vi "Data logger Default Paths.vi"(3 "Path Type":T1(ring)) -> (0 "Path":path)   [LabVIEW 2014]
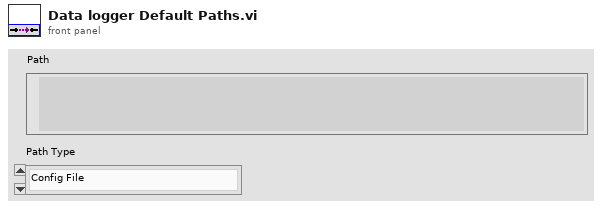
[diagram p1: front panel]
types:
  T1 = enum16{"Config File", "Image File", "Word Template", "Release Note", "Help HTML", "Help Word", "Error List", "Excel Template", "CSV Template", "Tray Icon"}
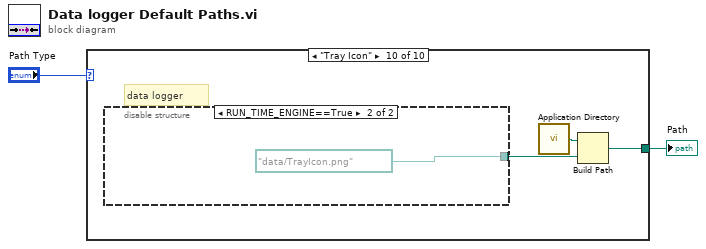
[diagram p0: block diagram]
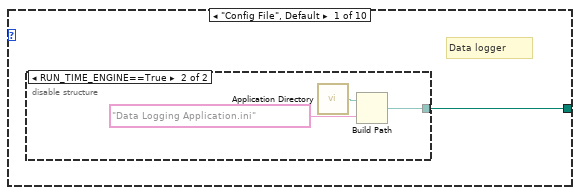
[diagram p2: hidden frame]
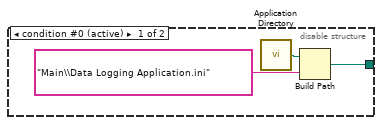
[diagram p3: hidden frame]
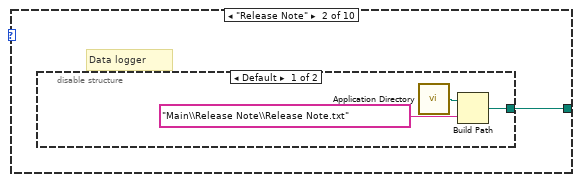
[diagram p4: hidden frame]
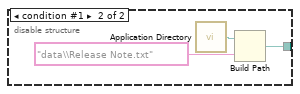
[diagram p5: hidden frame]
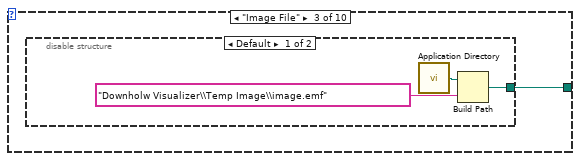
[diagram p6: hidden frame]
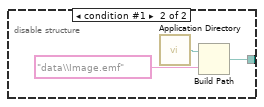
[diagram p7: hidden frame]
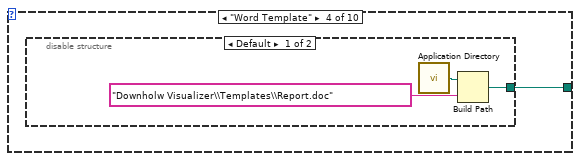
[diagram p8: hidden frame]
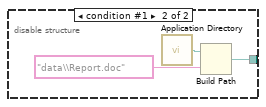
[diagram p9: hidden frame]
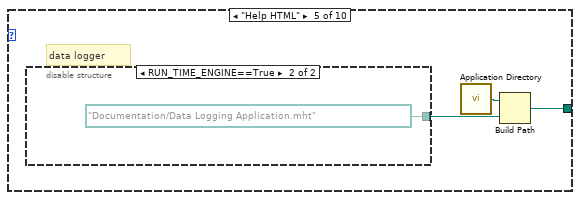
[diagram p10: hidden frame]
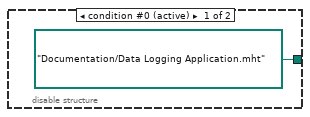
[diagram p11: hidden frame]
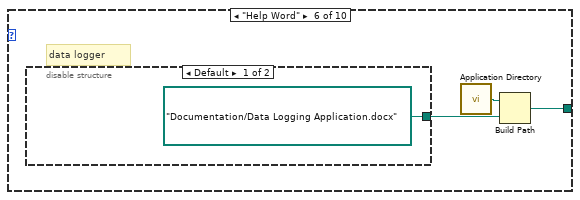
[diagram p12: hidden frame]
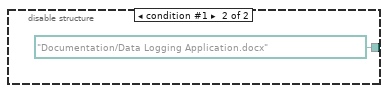
[diagram p13: hidden frame]
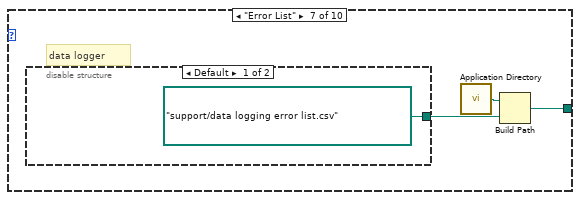
[diagram p14: hidden frame]
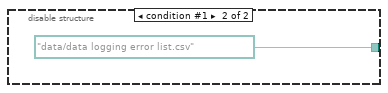
[diagram p15: hidden frame]
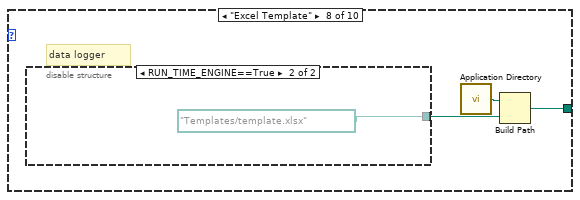
[diagram p16: hidden frame]
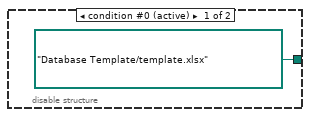
[diagram p17: hidden frame]
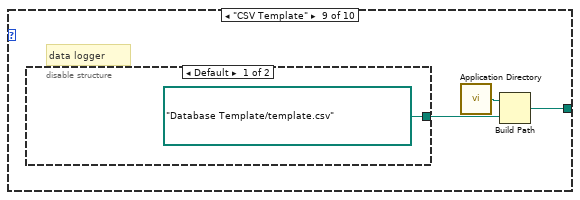
[diagram p18: hidden frame]
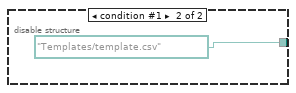
[diagram p19: hidden frame]
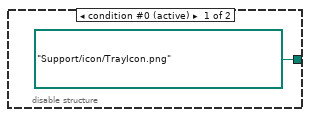
[diagram p20: hidden frame]
diagram:
  n1 = case shown="\"Tray Icon\"" "Path Type" {
    tunnel: [w3 w10 w17 w24 w31 w36 w41 w46 w51 w56] -> w1
    frame "Config File", Default {
      # "Data logger"
      n2 = disable-structure shown="RUN_TIME_ENGINE==True" {
        disable-tunnel: [w4 w7] -> w3
        frame condition #0 (active) {
          n3 = call <vilib>:"Application Directory.vi"() -> ("Application Directory"=w6:path)
          n4 = Build Path(base path=w6, name or relative path="Main\\Data Logging Application.ini") -> (appended path=w4:path)
        }
        frame condition #1 {
          n5 = call <vilib>:"Application Directory.vi"() -> ("Application Directory"=w9:path)
          n6 = Build Path(base path=w9, name or relative path="Data Logging Application.ini") -> (appended path=w7:path)
        }
      }
    }
    frame "Release Note" {
      # "Data logger"
      n7 = disable-structure shown="Default" {
        disable-tunnel: [w11 w14] -> w10
        frame condition #0 (active) {
          n8 = call <vilib>:"Application Directory.vi"() -> ("Application Directory"=w13:path)
          n9 = Build Path(base path=w13, name or relative path="Main\\Release Note\\Release Note.txt") -> (appended path=w11:path)
        }
        frame condition #1 {
          n10 = call <vilib>:"Application Directory.vi"() -> ("Application Directory"=w16:path)
          n11 = Build Path(base path=w16, name or relative path="data\\Release Note.txt") -> (appended path=w14:path)
        }
      }
    }
    frame "Image File" {
      n12 = disable-structure shown="Default" {
        disable-tunnel: [w19 w21] -> w17
        frame condition #0 (active) {
          n13 = call <vilib>:"Application Directory.vi"() -> ("Application Directory"=w20:path)
          n14 = Build Path(base path=w20, name or relative path="Downholw Visualizer\\Temp Image\\image.emf") -> (appended path=w19:path)
        }
        frame condition #1 {
          n15 = call <vilib>:"Application Directory.vi"() -> ("Application Directory"=w23:path)
          n16 = Build Path(base path=w23, name or relative path="data\\Image.emf") -> (appended path=w21:path)
        }
      }
    }
    frame "Word Template" {
      n17 = disable-structure shown="Default" {
        disable-tunnel: [w25 w28] -> w24
        frame condition #0 (active) {
          n18 = call <vilib>:"Application Directory.vi"() -> ("Application Directory"=w27:path)
          n19 = Build Path(base path=w27, name or relative path="Downholw Visualizer\\Templates\\Report.doc") -> (appended path=w25:path)
        }
        frame condition #1 {
          n20 = call <vilib>:"Application Directory.vi"() -> ("Application Directory"=w30:path)
          n21 = Build Path(base path=w30, name or relative path="data\\Report.doc") -> (appended path=w28:path)
        }
      }
    }
    frame "Help HTML" {
      # "data logger"
      n22 = disable-structure shown="RUN_TIME_ENGINE==True" {
        disable-tunnel: [path "Documentation/Data Logging Application.mht" path "Documentation/Data Logging Application.mht"] -> w32
        frame condition #0 (active) {
        }
        frame condition #1 {
        }
      }
      n23 = call <vilib>:"Application Directory.vi"() -> ("Application Directory"=w33:path)
      n24 = Build Path(base path=w33, name or relative path=w32) -> (appended path=w31:path)
    }
    frame "Help Word" {
      # "data logger"
      n25 = disable-structure shown="Default" {
        disable-tunnel: [path "Documentation/Data Logging Application.docx" path "Documentation/Data Logging Application.docx"] -> w37
        frame condition #0 (active) {
        }
        frame condition #1 {
        }
      }
      n26 = call <vilib>:"Application Directory.vi"() -> ("Application Directory"=w38:path)
      n27 = Build Path(base path=w38, name or relative path=w37) -> (appended path=w36:path)
    }
    frame "Error List" {
      # "data logger"
      n28 = disable-structure shown="Default" {
        disable-tunnel: [path "support/data logging error list.csv" path "data/data logging error list.csv"] -> w42
        frame condition #0 (active) {
        }
        frame condition #1 {
        }
      }
      n29 = call <vilib>:"Application Directory.vi"() -> ("Application Directory"=w43:path)
      n30 = Build Path(base path=w43, name or relative path=w42) -> (appended path=w41:path)
    }
    frame "Excel Template" {
      # "data logger"
      n31 = disable-structure shown="RUN_TIME_ENGINE==True" {
        disable-tunnel: [path "Database Template/template.xlsx" path "Templates/template.xlsx"] -> w47
        frame condition #0 (active) {
        }
        frame condition #1 {
        }
      }
      n32 = call <vilib>:"Application Directory.vi"() -> ("Application Directory"=w48:path)
      n33 = Build Path(base path=w48, name or relative path=w47) -> (appended path=w46:path)
    }
    frame "CSV Template" {
      # "data logger"
      n34 = disable-structure shown="Default" {
        disable-tunnel: [path "Database Template/template.csv" path "Templates/template.csv"] -> w52
        frame condition #0 (active) {
        }
        frame condition #1 {
        }
      }
      n35 = call <vilib>:"Application Directory.vi"() -> ("Application Directory"=w53:path)
      n36 = Build Path(base path=w53, name or relative path=w52) -> (appended path=w51:path)
    }
    frame "Tray Icon" {
      # "data logger"
      n37 = disable-structure shown="RUN_TIME_ENGINE==True" {
        disable-tunnel: [path "Support/icon/TrayIcon.png" path "data/TrayIcon.png"] -> w57
        frame condition #0 (active) {
        }
        frame condition #1 {
        }
      }
      n38 = call <vilib>:"Application Directory.vi"() -> ("Application Directory"=w58:path)
      n39 = Build Path(base path=w58, name or relative path=w57) -> (appended path=w56:path)
    }
  }
  "Path" <- w1
